vi "Proyecto VISA (PID).vi"() -> ()   [LabVIEW 2013]
uses:
  <vilib>/userdefined/High Color/IMAQdx.ctl
  <vilib>/Instr/_visa.llb/VISA Configure Serial Port (Instr).vi
  <vilib>/vision/driver/NI_Vision_Acquisition_Software.lvlib
  <vilib>/vision/NI_Vision_Development_Module.lvlib
  <vilib>/addons/control/pid/NI_PID_autopid.lvlib
panel:
  in  "output range 4":cluster{"output high":dbl, "output low":dbl}={"output high"=100.0, "output low"=-100.0} {"output low" format="%.2f"; "output high" format="%.2f"}
  in  "output range 3":cluster{"output high":dbl, "output low":dbl}={"output high"=100.0, "output low"=-100.0} {"output low" format="%.2f"; "output high" format="%.2f"}
  in  "output range 2":cluster{"output high":dbl, "output low":dbl}={"output high"=100.0, "output low"=-100.0} {"output low" format="%.2f"; "output high" format="%.2f"}
  in  "output range":cluster{"output high":dbl, "output low":dbl}={"output high"=100.0, "output low"=-100.0} {"output low" format="%.2f"; "output high" format="%.2f"}
  in  "dt (s)":dbl=-1.0 format="%.3f"
  in  "PID gains":T1={"proportional gain (Kc)"=1.0, "integral time (Ti, min)"=0.01, "derivative time (Td, min)"=0.0} {"derivative time (Td, min)" format="%.8f"; "integral time (Ti, min)" format="%.8f"; "proportional gain (Kc)" format="%.8f"}
  in  "data bits (8)":u16=8 min=5 max=8 step=1
  out "X":string
  in  "Pos. X":u8
  in  "Pos. Y":u8
  in  "baud rate (9600)":u32=9600
  in  "VISA resource name":refnum<visa-resource-name>
  out "Y":string
  in  "Centro de Y":dbl
  in  "Centro de X":dbl
  out "Pos. Servo Y":i32
  out "Pos. Servo X":i32
  out "Objeto Detectado":bool
  out "X":bool
  out "-Y":bool
  out "-X":bool
  out "Y":bool
  out "Valor de Y":sgl
  out "Valor de X":sgl
  in  "Color Plane":i32(ring)=1 items=["Red", "Green", "Blue", "Hue", "Saturation", "Luminance", "Value", "Intensity"]
  in  "stop":bool
  out "Image":T2(plugin-control)
  in  "Settings":T3={"Algorithm"=2, "Number of Matches Requested"=1, "Minimum Match Score"=800.0, "SubPixel Accuracy"=TRUE, "Rotation Angle Ranges"=[], "Show Search Area"=FALSE, "Show Result"=TRUE} {"Rotation Angle Ranges"."End" format="%.1f"; "Rotation Angle Ranges"."Start" format="%.1f"; "Minimum Match Score" min=0 max=1000 format="%.2f"; "Number of Matches Requested" min=1; "Algorithm" items=["All", "Low Discrepancy Sampling", "Grayscale Value Pyramid", "Gradients Pyramid"]}
  in  "Search Rect":T4={"Left"=0, "Top"=0, "Right"=2147483647, "Bottom"=2147483647, "Rotation"=0.0} {"Rotation" format="%.2f"; "Left" scale=0.0..1024.0; "Right" scale=0.0..1024.0}
  in  "File Path":path
  # "Valores en servo X 45°\nSi servo>45°=Abajo\nSi servo<45°=Arriba"
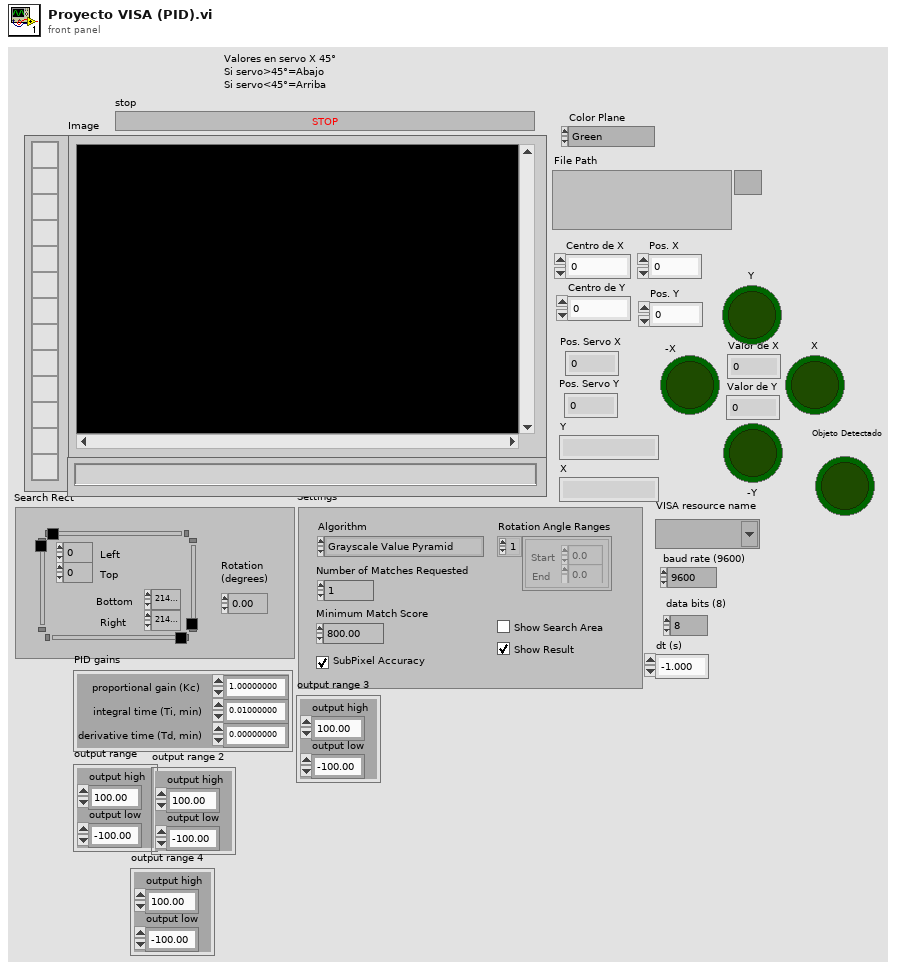
[diagram p1: front panel]
types:
  T1 = cluster{"proportional gain (Kc)":dbl, "integral time (Ti, min)":dbl, "derivative time (Td, min)":dbl}
  T2 = typedef "IMAQ Image.ctl" = refnum<image>
  T3 = cluster{"Algorithm":i32, "Number of Matches Requested":i32, "Minimum Match Score":sgl, "SubPixel Accuracy":bool, "Rotation Angle Ranges":cluster{"Start":sgl, "End":sgl}[], "Show Search Area":bool, "Show Result":bool}
  T4 = typedef "IMAQ Rectangle" = cluster{"Left":i32, "Top":i32, "Right":i32, "Bottom":i32, "Rotation":dbl}
  T5 = typedef "IMAQdx.ctl" = refnum<k21>
  T6 = cluster{"Position":cluster{"x":sgl, "y":sgl}, "Angle":sgl, "Scale":sgl, "Score":sgl, "Bounding Box":cluster{"x":sgl, "y":sgl}[]}[]
  T7 = cluster{"Matches (pixel)[0]":cluster{"Position":cluster{"x":sgl, "y":sgl}, "Angle":sgl, "Scale":sgl, "Score":sgl, "Bounding Box":cluster{"x":sgl, "y":sgl}[]}, "Matches (pixel)[1]":cluster{"Position":cluster{"x":sgl, "y":sgl}, "Angle":sgl, "Scale":sgl, "Score":sgl, "Bounding Box":cluster{"x":sgl, "y":sgl}[]}, "Matches (pixel)[2]":cluster{"Position":cluster{"x":sgl, "y":sgl}, "Angle":sgl, "Scale":sgl, "Score":sgl, "Bounding Box":cluster{"x":sgl, "y":sgl}[]}, "Matches (pixel)[3]":cluster{"Position":cluster{"x":sgl, "y":sgl}, "Angle":sgl, "Scale":sgl, "Score":sgl, "Bounding Box":cluster{"x":sgl, "y":sgl}[]}, "Matches (pixel)[4]":cluster{"Position":cluster{"x":sgl, "y":sgl}, "Angle":sgl, "Scale":sgl, "Score":sgl, "Bounding Box":cluster{"x":sgl, "y":sgl}[]}, "Matches (pixel)[5]":cluster{"Position":cluster{"x":sgl, "y":sgl}, "Angle":sgl, "Scale":sgl, "Score":sgl, "Bounding Box":cluster{"x":sgl, "y":sgl}[]}, "Matches (pixel)[6]":cluster{"Position":cluster{"x":sgl, "y":sgl}, "Angle":sgl, "Scale":sgl, "Score":sgl, "Bounding Box":cluster{"x":sgl, "y":sgl}[]}, "Matches (pixel)[7]":cluster{"Position":cluster{"x":sgl, "y":sgl}, "Angle":sgl, "Scale":sgl, "Score":sgl, "Bounding Box":cluster{"x":sgl, "y":sgl}[]}, "Matches (pixel)[8]":cluster{"Position":cluster{"x":sgl, "y":sgl}, "Angle":sgl, "Scale":sgl, "Score":sgl, "Bounding Box":cluster{"x":sgl, "y":sgl}[]}}
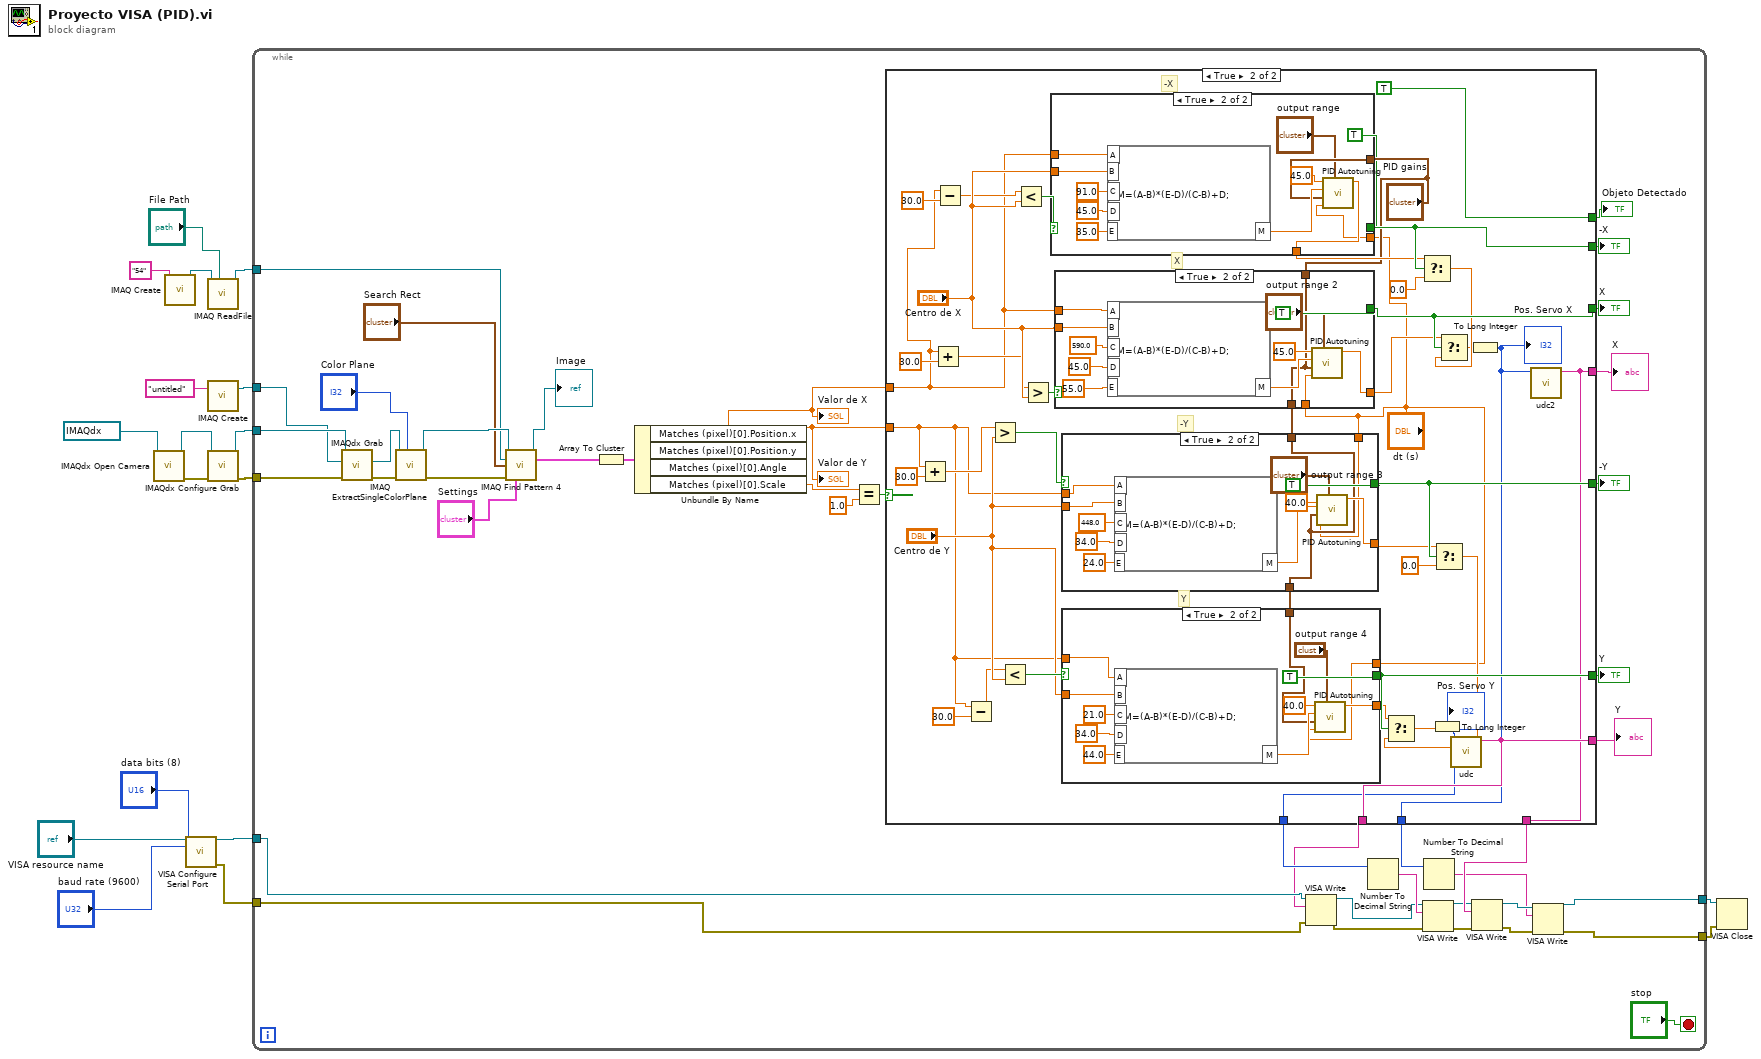
[diagram p0: block diagram]
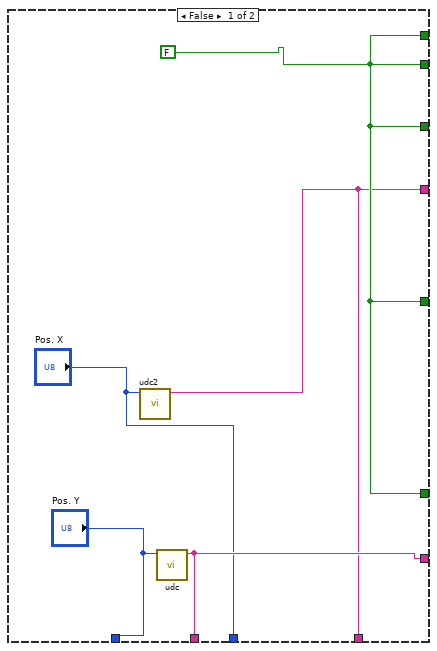
[diagram p2: hidden frame]
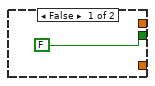
[diagram p3: hidden frame]
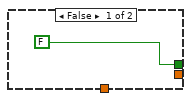
[diagram p4: hidden frame]
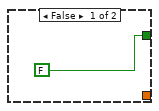
[diagram p5: hidden frame]
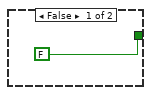
[diagram p6: hidden frame]
diagram:
  n1 = call <vilib>:"IMAQdx Open Camera.vi"("Session In"=T5 "cam1") -> ("error out"=w18:errorcluster, "Session Out"=w17:T5)  [unwired: 9 in]
  n2 = call "IMAQ Create"("Image Name"="54") -> ("New Image"=w10:T2)  [unwired: 4 in, 1 out]
  n3 = call-poly "VISA Configure Serial Port"("VISA resource name"="VISA resource name", "baud rate (9600)"="baud rate (9600)", "data bits (8)"="data bits (8)") -> ("VISA resource name out"=w4:refnum<visa-resource-name>, "error out"=w5:errorcluster)  [unwired: 11 in]
  n4 = call "IMAQ ReadFile"("File Path"="File Path", "Image"=w10) -> ("Image Out"=w9:T2)  [unwired: 5 in, 4 out]
  n5 = call "IMAQ Create"("Image Name"="untitled") -> ("New Image"=w12:T2)  [unwired: 4 in, 1 out]
  n6 = call <vilib>:"IMAQdx Configure Grab.vi"("error in"=w18, "Session In"=w17) -> ("error out"=w15:errorcluster, "Session Out"=w16:T5)  [unwired: 8 in]
  n7 = while {
    tunnel: w16 -> [w61]
    tunnel: w15 -> [w60]
    tunnel: w12 -> [w56]
    tunnel: w9 -> [w54]
    tunnel: w5 -> [w33]
    tunnel: w4 -> [w34]
    tunnel: [w20] -> w2
    tunnel: [w19] -> w1
    stop <- "stop" stop-if-true
    n8 = call <vilib>:"IMAQdx Grab.vi"("error in"=w60, "Image In"=w56, "Session In"=w61) -> ("error out"=w59:errorcluster, "Image Out"=w55:T2)  [unwired: 5 in, 2 out]
    n9 = call "IMAQ ExtractSingleColorPlane"("Color Plane"="Color Plane", "error in (no error)"=w59, "Image Src"=w55) -> ("error out"=w57:errorcluster, "Image Dst Out"=w58:T2)  [unwired: 7 in]
    n10 = call "IMAQ Find Pattern 4"("Image"=w58, "Template"=w54, "Search Rect"="Search Rect", "error in"=w57, "Settings"="Settings") -> ("Image Out"=→"Image":T2, "Matches (pixel)"=w48:T6)  [unwired: 4 in, 5 out]
    n11 = Array To Cluster(array=w48) -> (cluster=w49:T7)
    n12 = Unbundle By Name(w49) -> ("Matches (pixel)[0].Position.x"=w47:sgl, "Matches (pixel)[0].Position.y"=w46:sgl, "Matches (pixel)[0].Scale"=w45:sgl)  [unwired: 1 out]
    "Valor de X" <- w47
    "Valor de Y" <- w46
    n13 = Equal?(x=w45, y=sgl 1.0) -> (x = y?=w43:bool)
    n14 = case shown="True" w43 {
      tunnel: w47 -> [_ w83]
      tunnel: w46 -> [_ w78]
      tunnel: [w66 TRUE] -> w42
      tunnel: [w66 w97] -> w41
      tunnel: [w66 w100] -> w40
      tunnel: [w66 w94] -> w39
      tunnel: [w66 w91] -> w38
      tunnel: ["Pos. Y" w72] -> w36
      tunnel: [w65 w77] -> w35
      tunnel: [w65 w77] -> w32
      tunnel: [w63 w76] -> w31
      tunnel: [w63 w76] -> w30
      tunnel: ["Pos. X" w74] -> w29
      frame False {
        w66 = FALSE
        n15 = call "udc2.vi"("Numeric"="Pos. X") -> ("s? t:f"=w63:string)  [unwired: 10 in]
        n16 = call "udc.vi"("Numeric"="Pos. Y") -> ("s? t:f"=w65:string)  [unwired: 10 in]
      }
      frame True {
        # "X"
        # "-X"
        # "Y"
        # "-Y"
        n17 = Add(x=w78, y=30.0) -> (x+y=w80:dbl)
        n18 = Add(x=w83, y=30.0) -> (x+y=w87:dbl)
        n19 = Subtract(x=w83, y=30.0) -> (x-y=w85:dbl)
        n20 = Subtract(x=w78, y=30.0) -> (x-y=w82:dbl)
        n21 = Greater?(x=w80, y="Centro de Y") -> (0:w104:bool)
        n22 = Less?(x=w82, y="Centro de Y") -> (x < y?=w102:bool)
        n23 = Less?(x=w85, y="Centro de X") -> (x < y?=w103:bool)
        n24 = Greater?(x=w87, y="Centro de X") -> (0:w105:bool)
        n25 = case shown="True" w103 {
          tunnel: [FALSE TRUE] -> w100
          tunnel: "Centro de X" -> [_ w129]
          tunnel: w83 -> [_ w128]
          tunnel: [_ w123] -> w99
          tunnel: "PID gains" -> [_ w122]
          tunnel: "dt (s)" -> [_ w121]
          frame False {
          }
          frame True {
            n26 = formula code="M=(A-B)*(E-D)/(C-B)+D;"("A"=w128, "B"=w129, "C"=91.0 ("input variable"), "D"=45.0 ("input variable"), "E"=35.0 ("input variable")) -> ("M"=w124:dbl)
            n27 = call <vilib>:"PID Autotuning.vi"("output range"="output range", "dt (s)"=w121, "PID gains"=w122, "process variable"=w124, "setpoint"=45.0) -> ("output"=w123:dbl)  [unwired: 3 in, 3 out]
          }
        }
        n28 = case shown="True" w105 {
          tunnel: [FALSE TRUE] -> w97
          tunnel: w83 -> [_ w153]
          tunnel: "Centro de X" -> [_ w152]
          tunnel: [_ w149] -> w96
          tunnel: "PID gains" -> [_ w146]
          tunnel: "dt (s)" -> [_ w148]
          tunnel: [_ w146] -> w70
          frame False {
          }
          frame True {
            n29 = formula code="M=(A-B)*(E-D)/(C-B)+D;"("A"=w153, "B"=w152, "C"=590.0 ("input variable"), "D"=45.0 ("input variable"), "E"=55.0 ("input variable")) -> ("M"=w150:dbl)
            n30 = call <vilib>:"PID Autotuning.vi"("output range"="output range 2", "dt (s)"=w148, "PID gains"=w146, "process variable"=w150, "setpoint"=45.0) -> ("output"=w149:dbl)  [unwired: 3 in, 3 out]
          }
        }
        n31 = case shown="True" w104 {
          tunnel: [FALSE TRUE] -> w94
          tunnel: "Centro de Y" -> [_ w142]
          tunnel: [_ w135] -> w93
          tunnel: w78 -> [_ w139]
          tunnel: w70 -> [_ w134]
          tunnel: [_ w134] -> w68
          tunnel: "dt (s)" -> [_ w133]
          frame False {
          }
          frame True {
            n32 = formula code="M=(A-B)*(E-D)/(C-B)+D;"("A"=w139, "B"=w142, "C"=448.0 ("input variable"), "D"=34.0 ("input variable"), "E"=24.0 ("input variable")) -> ("M"=w136:dbl)
            n33 = call <vilib>:"PID Autotuning.vi"("output range"="output range 3", "dt (s)"=w133, "PID gains"=w134, "process variable"=w136, "setpoint"=40.0) -> ("output"=w135:dbl)  [unwired: 3 in, 3 out]
          }
        }
        n34 = case shown="True" w102 {
          tunnel: [FALSE TRUE] -> w91
          tunnel: "Centro de Y" -> [_ w116]
          tunnel: w78 -> [_ w115]
          tunnel: [_ w110] -> w69
          tunnel: w68 -> [_ w108]
          tunnel: "dt (s)" -> [_ w107]
          frame False {
          }
          frame True {
            n35 = formula code="M=(A-B)*(E-D)/(C-B)+D;"("A"=w115, "B"=w116, "C"=21.0 ("input variable"), "D"=34.0 ("input variable"), "E"=44.0 ("input variable")) -> ("M"=w111:dbl)
            n36 = call <vilib>:"PID Autotuning.vi"("output range"="output range 4", "dt (s)"=w107, "PID gains"=w108, "process variable"=w111, "setpoint"=40.0) -> ("output"=w110:dbl)  [unwired: 3 in, 3 out]
          }
        }
        n37 = Select(t=w99, s=w100, f=0.0) -> (s? t:f=w95:dbl)
        n38 = Select(t=w93, s=w94, f=0.0) -> (s? t:f=w90:dbl)
        n39 = Select(t=w69, s=w91, f=w90) -> (s? t:f=w73:dbl)
        n40 = To Long Integer(number=w73) -> (32bit integer=w72:i32)
        "Pos. Servo Y" <- w72
        n41 = Select(t=w96, s=w97, f=w95) -> (s? t:f=w75:dbl)
        n42 = call "udc.vi"("Numeric"=w72) -> ("s? t:f"=w77:string)  [unwired: 10 in]
        n43 = To Long Integer(number=w75) -> (32bit integer=w74:i32)
        "Pos. Servo X" <- w74
        n44 = call "udc2.vi"("Numeric"=w74) -> ("s? t:f"=w76:string)  [unwired: 10 in]
      }
    }
    "Objeto Detectado" <- w42
    "X" <- w41
    "-X" <- w40
    "Y" <- w38
    "-Y" <- w39
    "Y" <- w35
    "X" <- w31
    n45 = VISA Write(VISA resource name=w34, write buffer=w32, error in (no error)=w33) -> (VISA resource name out=w27:refnum<visa-resource-name>, error out=w21:errorcluster)  [unwired: 1 out]
    n46 = Number To Decimal String(number=w36) -> (decimal integer string=w28:string)  [unwired: 1 in]
    n47 = VISA Write(VISA resource name=w27, write buffer=w28, error in (no error)=w21) -> (VISA resource name out=w25:refnum<visa-resource-name>, error out=w24:errorcluster)  [unwired: 1 out]
    n48 = Number To Decimal String(number=w29) -> (decimal integer string=w22:string)  [unwired: 1 in]
    n49 = VISA Write(VISA resource name=w25, write buffer=w30, error in (no error)=w24) -> (VISA resource name out=w26:refnum<visa-resource-name>, error out=w23:errorcluster)  [unwired: 1 out]
    n50 = VISA Write(VISA resource name=w26, write buffer=w22, error in (no error)=w23) -> (VISA resource name out=w20:refnum<visa-resource-name>, error out=w19:errorcluster)  [unwired: 1 out]
  }
  n51 = VISA Close(VISA resource name=w2, error in (no error)=w1) -> ()  [unwired: 1 out]
